vi "Read Arduino Analog Pins.vi"(0 "Arduino Resource In":T1={"VISA resource"="", "Board Type"=enum."Uno", "Connection Type"=enum."USB / Serial", "Bytes Per Packet (15)"=15}, 2 "Mean Sample Length":i32=10, 5 "Arduino Error In":errorcluster, 7 "Photoresistor Sample Length":i32=10) -> (11 "Sonar Rear Left (Meters)":dbl, 13 "Sonar Rear Right (Meters)":dbl, 14 "Arduino Resource Out":T1={"VISA resource"="COM11", "Board Type"=enum."Uno", "Connection Type"=enum."USB / Serial", "Bytes Per Packet (15)"=15}, 15 "Sonar Front Left (Meters)":dbl, 16 "Sonar Front Center (Meters)":dbl, 17 "Sonar Front Right (Meters)":dbl, 18 "Photoresistor Voltage":dbl(knob) scale=0.0..5.0, 19 "Arduino Error Out":errorcluster)   [LabVIEW 2011]
uses:
  <vilib>/LabVIEW Interface for Arduino/Type Defs/Arduino Resource.ctl
  <vilib>/LabVIEW Interface for Arduino/Type Defs/Board Type.ctl
  <vilib>/express/express arith-compare/Formula/XNode/ExpressFormulaBlockNode.xnode
  <vilib>/LabVIEW Interface for Arduino/LabVIEW Interface for Arduino.lvlib
panel:
  out "V_Pin4":dbl(slide) scale=0.0..10.0 scale format="%_4g"
  out "V_Pin5":dbl(slide) scale=0.0..10.0 scale format="%_4g"
  out "V_Pin3":dbl(slide) scale=0.0..10.0 scale format="%_4g"
  out "V_Pin2":dbl(slide) scale=0.0..10.0 scale format="%_4g"
  out "V_Pin1":dbl(slide) scale=0.0..10.0 scale format="%_4g"
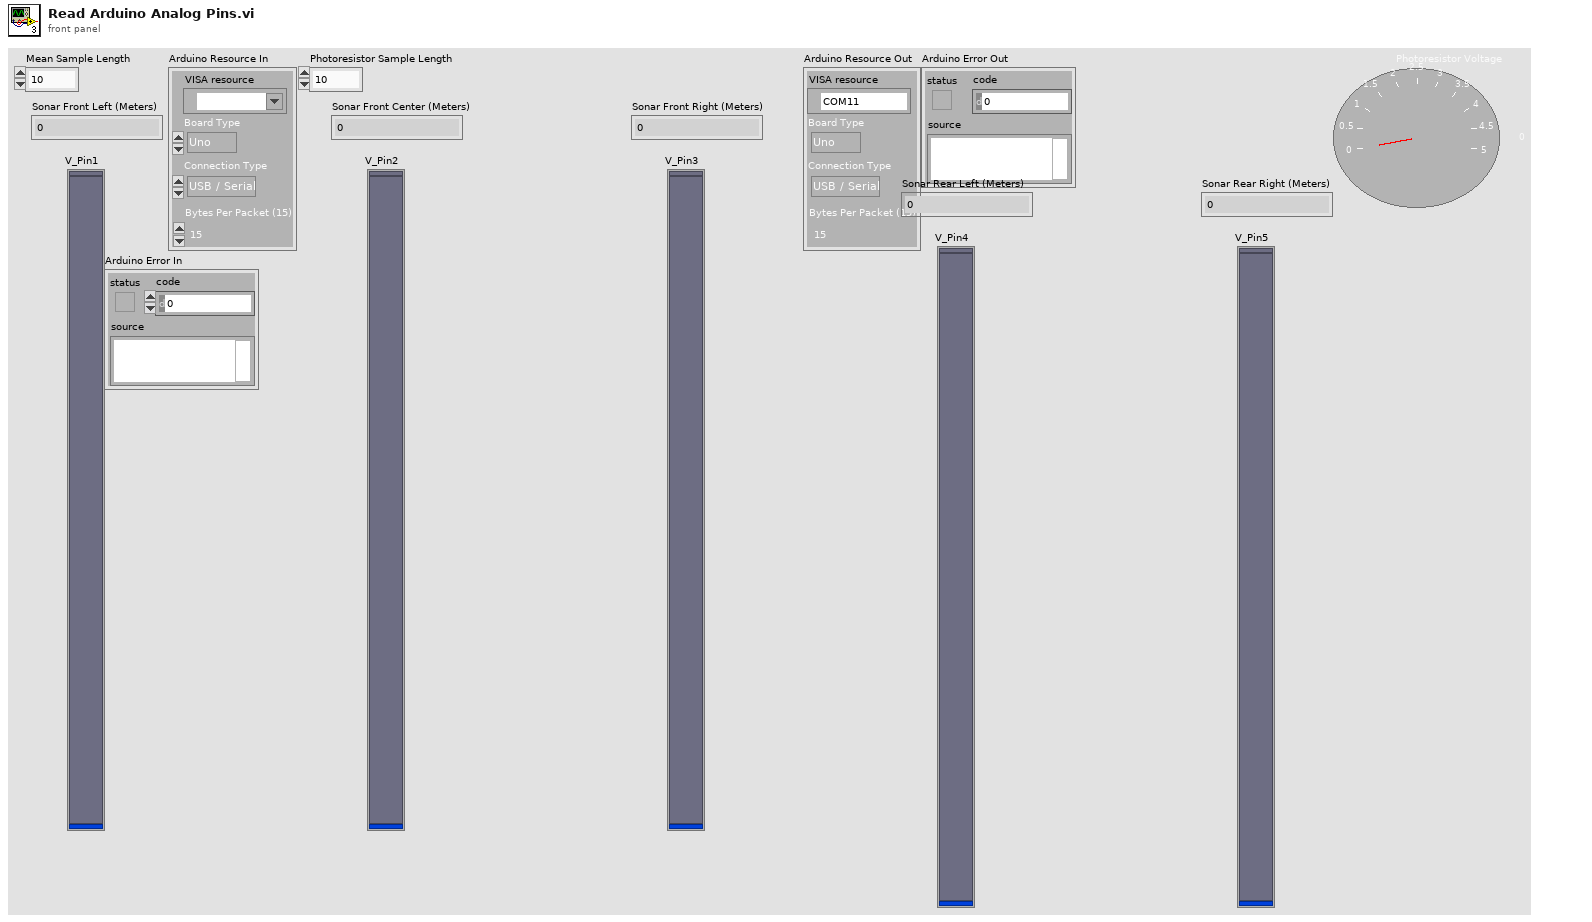
[diagram p1: front panel]
types:
  T1 = typedef "LabVIEW Interface for Arduino.lvlib/Arduino Resource.ctl" = cluster{"VISA resource":refnum<visa-resource-name>, "Board Type":T2, "Connection Type":enum8{"USB / Serial"}, "Bytes Per Packet (15)":u8}
  T2 = typedef "LabVIEW Interface for Arduino.lvlib/Board Type.ctl" = enum16{"Uno", "Dimuelanove w/Atmega 328", "Mega 2560"}
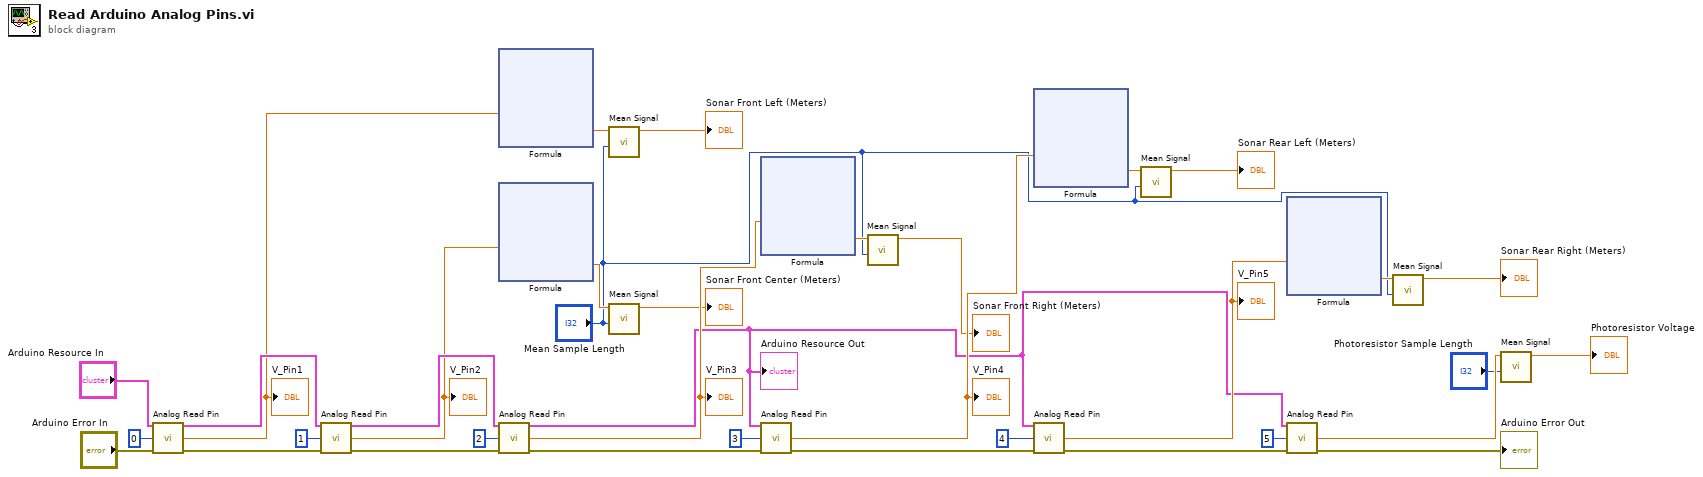
[diagram p0: block diagram]
diagram:
  n1 = call <vilib>:"Analog Read Pin.vi"("Arduino Resource"="Arduino Resource In", "Analog Input Pin (0)"=u8 0, "error in"="Arduino Error In") -> ("Arduino Resource"=w35:T1, "Voltage"=w23:dbl, "error out"=w32:errorcluster)  [unwired: 10 in]
  "V_Pin1" <- w23
  n2 = call <vilib>:"Analog Read Pin.vi"("Arduino Resource"=w35, "Analog Input Pin (0)"=u8 1, "error in"=w32) -> ("Arduino Resource"=w34:T1, "Voltage"=w22:dbl, "error out"=w33:errorcluster)  [unwired: 10 in]
  "V_Pin2" <- w22
  n3 = xnode "Formula"("Vin"=w23) -> ("Result"=w18:dbl)  [unwired: 1 in, 1 out]
  n4 = xnode "Formula"("Vin"=w22) -> ("Result"=w12:dbl)  [unwired: 1 in, 1 out]
  n5 = call <vilib>:"Analog Read Pin.vi"("Arduino Resource"=w34, "Analog Input Pin (0)"=u8 2, "error in"=w33) -> ("Arduino Resource"=w5:T1, "Voltage"=w20:dbl, "error out"=w24:errorcluster)  [unwired: 10 in]
  "V_Pin3" <- w20
  "Arduino Resource Out" <- w5
  n6 = call "Mean Signal.vi"("sample length"="Mean Sample Length", "Signal In"=w18) -> ("Signal Out"=→"Sonar Front Left (Meters)":dbl)  [unwired: 9 in]
  n7 = call "Mean Signal.vi"("sample length"="Mean Sample Length", "Signal In"=w12) -> ("Signal Out"=→"Sonar Front Center (Meters)":dbl)  [unwired: 9 in]
  n8 = xnode "Formula"("Vin"=w20) -> ("Result"=w11:dbl)  [unwired: 1 in, 1 out]
  n9 = call <vilib>:"Analog Read Pin.vi"("Arduino Resource"=w5, "Analog Input Pin (0)"=u8 3, "error in"=w24) -> ("Voltage"=w19:dbl, "error out"=w25:errorcluster)  [unwired: 10 in, 1 out]
  "V_Pin4" <- w19
  n10 = call "Mean Signal.vi"("sample length"="Mean Sample Length", "Signal In"=w11) -> ("Signal Out"=→"Sonar Front Right (Meters)":dbl)  [unwired: 9 in]
  n11 = xnode "Formula"("Vin"=w19) -> ("Result"=w10:dbl)  [unwired: 1 in, 1 out]
  n12 = call <vilib>:"Analog Read Pin.vi"("Arduino Resource"=w5, "Analog Input Pin (0)"=u8 4, "error in"=w25) -> ("Voltage"=w21:dbl, "error out"=w7:errorcluster)  [unwired: 10 in, 1 out]
  "V_Pin5" <- w21
  n13 = call "Mean Signal.vi"("sample length"="Mean Sample Length", "Signal In"=w10) -> ("Signal Out"=→"Sonar Rear Left (Meters)":dbl)  [unwired: 9 in]
  n14 = xnode "Formula"("Vin"=w21) -> ("Result"=w9:dbl)  [unwired: 1 in, 1 out]
  n15 = call <vilib>:"Analog Read Pin.vi"("Arduino Resource"=w5, "Analog Input Pin (0)"=u8 5, "error in"=w7) -> ("Voltage"=w3:dbl, "error out"=→"Arduino Error Out":errorcluster)  [unwired: 10 in, 1 out]
  n16 = call "Mean Signal.vi"("sample length"="Mean Sample Length", "Signal In"=w9) -> ("Signal Out"=→"Sonar Rear Right (Meters)":dbl)  [unwired: 9 in]
  n17 = call "Mean Signal.vi"("sample length"="Photoresistor Sample Length", "Signal In"=w3) -> ("Signal Out"=→"Photoresistor Voltage":dbl)  [unwired: 9 in]
